vi "HandleObservationSync_002.vi"(8 "error in (no error)":errorcluster, 11 "S4GUI in":refnum<class "S4GUI.lvclass">) -> (0 "error out":errorcluster, 3 "S4GUI out":refnum<class "S4GUI.lvclass">)   [LabVIEW 2018, in "S4GUI.lvclass"] (continued)
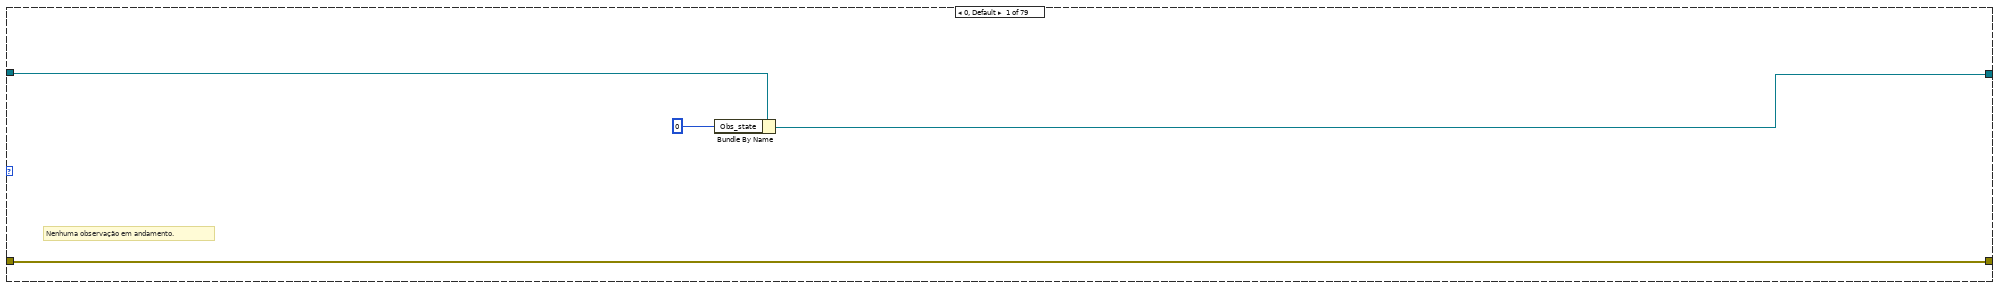
[diagram p2: hidden frame]
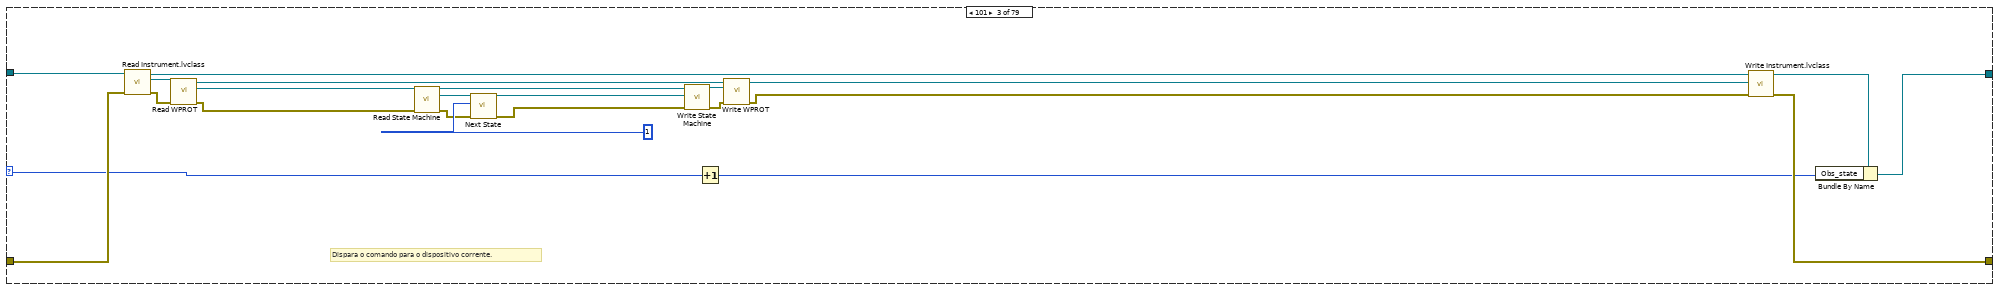
[diagram p4: hidden frame]
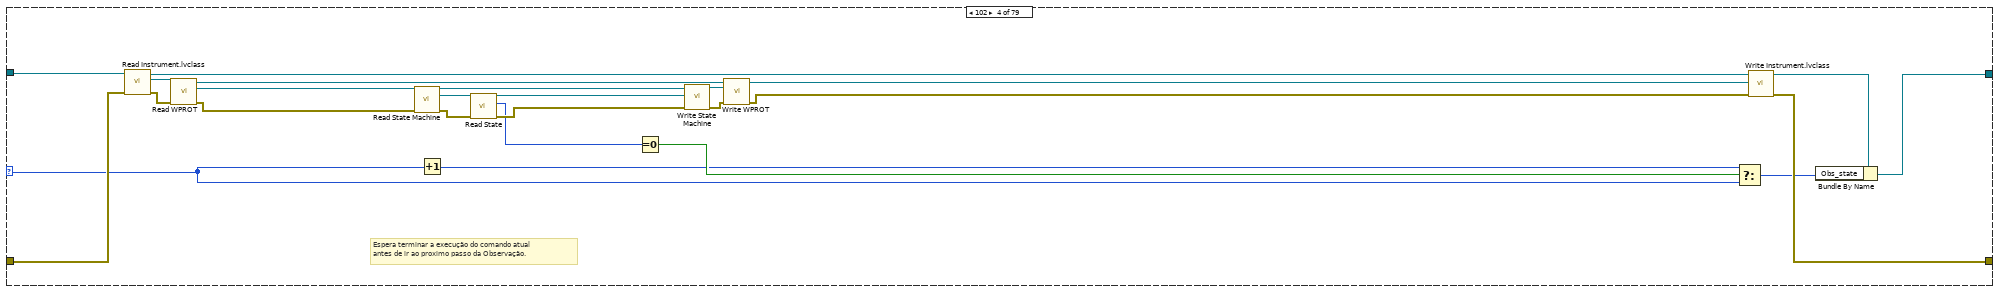
[diagram p5: hidden frame]
              n1811 = call-dynamic "Read Channel.vi"("error in (no error)"=w5159, "Acquisition in"=w5160) -> ("error out"=w5144:errorcluster, "Channel.lvclass"=w5146:refnum<class "Channel.lvclass">, "Acquisition out"=w5158:refnum<class "Acquisition.lvclass">)  [unwired: 7 in]
              n1812 = call-dynamic "Read wait_expose.vi"("error in (no error)"=w5144, "Channel in"=w5146) -> ("error out"=w5143:errorcluster, "wait_expose"=w5142:bool, "Channel out"=w5145:refnum<class "Channel.lvclass">)  [unwired: 7 in]
              n1813 = call-dynamic "Read State Machine.vi"("error in (no error)"=w5143, "Device in"=w5145) -> ("error out"=w5150:errorcluster, "State Machine.lvclass"=w5152:refnum<class "State Machine.lvclass">, "Device out"=w5154:refnum<class "Channel.lvclass">)  [unwired: 7 in]
              n1814 = call-dynamic "Read State.vi"("error in (no error)"=w5150, "State Machine in"=w5152) -> ("error out"=w5149:errorcluster, "State"=w5147:i32, "State Machine out"=w5151:refnum<class "State Machine.lvclass">)  [unwired: 7 in]
              n1815 = Equal To 0?(x=w5147) -> (x = 0?=w5148:bool)
              n1816 = call-dynamic "Write State Machine.vi"("error in (no error)"=w5149, "State Machine.lvclass"=w5151, "Device in"=w5154) -> ("error out"=w5153:errorcluster, "Device out"=w5155:refnum<class "Channel.lvclass">)  [unwired: 7 in]
              n1817 = call-dynamic "Write Channel.vi"("error in (no error)"=w5153, "Channel.lvclass"=w5155, "Acquisition in"=w5158) -> ("error out"=w5156:errorcluster, "Acquisition out"=w5157:refnum<class "Acquisition.lvclass">)  [unwired: 7 in]
            }
          }
          n1818 = call "Write AcquisitionB.vi"("error in (no error)"=w5080, "Acquisition.lvclass"=w5082, "S4ACS_GUI in"=w5081) -> ("error out"=w5076:errorcluster, "S4ACS_GUI out"=w5075:refnum<class "S4GUI.lvclass">)  [unwired: 7 in]
          n1819 = call-dynamic "Read AcquisitionC.vi"("error in (no error)"=w5076, "S4ACS_GUI in"=w5075) -> ("error out"=w5058:errorcluster, "Acquisition.lvclass"=w5060:refnum<class "Acquisition.lvclass">, "S4ACS_GUI out"=w5078:refnum<class "S4GUI.lvclass">)  [unwired: 7 in]
          n1820 = call-dynamic "Read enabled.vi"("error in (no error)"=w5058, "Server in"=w5060) -> ("error out"=w5057:errorcluster, "enabled"=w5056:bool, "Server out"=w5059:refnum<class "Acquisition.lvclass">)  [unwired: 7 in]
          n1821 = case shown="True" w5056 {
            tunnel: [w5117 w5132] -> w5079
            tunnel: [w5118 w5131] -> w5077
            tunnel: w5059 -> [w5118 w5127]
            tunnel: w5057 -> [w5117 w5126]
            tunnel: [TRUE w5124] -> w5045
            tunnel: [FALSE ("expose") w5119] -> w5041
            frame False {
            }
            frame True {
              n1822 = call-dynamic "Read Channel.vi"("error in (no error)"=w5126, "Acquisition in"=w5127) -> ("error out"=w5121:errorcluster, "Channel.lvclass"=w5123:refnum<class "Channel.lvclass">, "Acquisition out"=w5130:refnum<class "Acquisition.lvclass">)  [unwired: 7 in]
              n1823 = call-dynamic "Read wait_expose.vi"("error in (no error)"=w5121, "Channel in"=w5123) -> ("error out"=w5120:errorcluster, "wait_expose"=w5119:bool, "Channel out"=w5122:refnum<class "Channel.lvclass">)  [unwired: 7 in]
              n1824 = call-dynamic "Read State Machine.vi"("error in (no error)"=w5120, "Device in"=w5122) -> ("error out"=w5128:errorcluster, "State Machine.lvclass"=w5136:refnum<class "State Machine.lvclass">, "Device out"=w5134:refnum<class "Channel.lvclass">)  [unwired: 7 in]
              n1825 = call-dynamic "Read State.vi"("error in (no error)"=w5128, "State Machine in"=w5136) -> ("error out"=w5129:errorcluster, "State"=w5125:i32, "State Machine out"=w5137:refnum<class "State Machine.lvclass">)  [unwired: 7 in]
              n1826 = Equal To 0?(x=w5125) -> (x = 0?=w5124:bool)
              n1827 = call-dynamic "Write State Machine.vi"("error in (no error)"=w5129, "State Machine.lvclass"=w5137, "Device in"=w5134) -> ("error out"=w5135:errorcluster, "Device out"=w5133:refnum<class "Channel.lvclass">)  [unwired: 7 in]
              n1828 = call-dynamic "Write Channel.vi"("error in (no error)"=w5135, "Channel.lvclass"=w5133, "Acquisition in"=w5130) -> ("error out"=w5132:errorcluster, "Acquisition out"=w5131:refnum<class "Acquisition.lvclass">)  [unwired: 7 in]
            }
          }
          n1829 = call-dynamic "Write AcquisitionC.vi"("error in (no error)"=w5079, "Acquisition.lvclass"=w5077, "S4ACS_GUI in"=w5078) -> ("error out"=w5055:errorcluster, "S4ACS_GUI out"=w5071:refnum<class "S4GUI.lvclass">)  [unwired: 7 in]
          n1830 = call-dynamic "Read AcquisitionD.vi"("error in (no error)"=w5055, "S4ACS_GUI in"=w5071) -> ("error out"=w5051:errorcluster, "Acquisition.lvclass"=w5054:refnum<class "Acquisition.lvclass">, "S4ACS_GUI out"=w5073:refnum<class "S4GUI.lvclass">)  [unwired: 7 in]
          n1831 = call-dynamic "Read enabled.vi"("error in (no error)"=w5051, "Server in"=w5054) -> ("error out"=w5052:errorcluster, "enabled"=w5050:bool, "Server out"=w5053:refnum<class "Acquisition.lvclass">)  [unwired: 7 in]
          n1832 = case shown="True" w5050 {
            tunnel: [w5095 w5113] -> w5074
            tunnel: [w5094 w5112] -> w5072
            tunnel: [TRUE w5102] -> w5044
            tunnel: w5053 -> [w5095 w5104]
            tunnel: w5052 -> [w5094 w5103]
            tunnel: [FALSE ("expose") w5096] -> w5040
            frame False {
            }
            frame True {
              n1833 = call-dynamic "Read Channel.vi"("error in (no error)"=w5103, "Acquisition in"=w5104) -> ("error out"=w5098:errorcluster, "Channel.lvclass"=w5100:refnum<class "Channel.lvclass">, "Acquisition out"=w5114:refnum<class "Acquisition.lvclass">)  [unwired: 7 in]
              n1834 = call-dynamic "Read wait_expose.vi"("error in (no error)"=w5098, "Channel in"=w5100) -> ("error out"=w5097:errorcluster, "wait_expose"=w5096:bool, "Channel out"=w5099:refnum<class "Channel.lvclass">)  [unwired: 7 in]
              n1835 = call-dynamic "Read State Machine.vi"("error in (no error)"=w5097, "Device in"=w5099) -> ("error out"=w5106:errorcluster, "State Machine.lvclass"=w5108:refnum<class "State Machine.lvclass">, "Device out"=w5110:refnum<class "Channel.lvclass">)  [unwired: 7 in]
              n1836 = call-dynamic "Read State.vi"("error in (no error)"=w5106, "State Machine in"=w5108) -> ("error out"=w5105:errorcluster, "State"=w5101:i32, "State Machine out"=w5107:refnum<class "State Machine.lvclass">)  [unwired: 7 in]
              n1837 = Equal To 0?(x=w5101) -> (x = 0?=w5102:bool)
              n1838 = call-dynamic "Write State Machine.vi"("error in (no error)"=w5105, "State Machine.lvclass"=w5107, "Device in"=w5110) -> ("error out"=w5109:errorcluster, "Device out"=w5111:refnum<class "Channel.lvclass">)  [unwired: 7 in]
              n1839 = call-dynamic "Write Channel.vi"("error in (no error)"=w5109, "Channel.lvclass"=w5111, "Acquisition in"=w5114) -> ("error out"=w5112:errorcluster, "Acquisition out"=w5113:refnum<class "Acquisition.lvclass">)  [unwired: 7 in]
            }
          }
          n1840 = call-dynamic "Write AcquisitionD.vi"("error in (no error)"=w5072, "Acquisition.lvclass"=w5074, "S4ACS_GUI in"=w5073) -> ("error out"=w5038:errorcluster, "S4ACS_GUI out"=w5039:refnum<class "S4GUI.lvclass">)  [unwired: 7 in]
          n1841 = Compound Arithmetic op=OR(w5043, w5042, w5041, w5040) -> ()  [unwired: 1 out]
          n1842 = Compound Arithmetic op=AND(w5047, w5046, w5045, w5044) -> (w5048:bool)
          n1843 = Increment(x=w5049) -> (x+1=w5037:u32)
          n1844 = Select(t=w5037, s=w5048, f=w5049) -> (s? t:f=w5085:u32)
          n1845 = Bundle By Name(cluster=w5039, "Obs_state"=w5085) -> (w5086:refnum<class "S4GUI.lvclass">)
        }
        frame 364 {
          n1846 = flat-sequence {
            tunnel: [w5197] -> w5185
            tunnel: w5186 -> [w5197]
            tunnel: [w5193] -> w5184
            frame #0 {
              # "Espera 2s desde que enviou o comando\nWRITE_HEADER_DATA para os ACS"
              n1847 = local read "time9"() -> (w5192:u32)
              n1848 = Tick Count (ms)() -> (millisecond timer value=w5196:u32)
              "time 10" <- w5196
              n1849 = Subtract(x=w5196, y=w5192) -> (x-y=w5195:u32)
              "delay 89" <- w5195
              n1850 = Greater?(x=w5195, y=u32 2000) -> (0:w5193:bool)
            }
          }
          n1851 = Increment(x=w5189) -> (x+1=w5188:u32)
          n1852 = Select(t=w5188, s=w5184, f=w5189) -> (s? t:f=w5190:u32)
          n1853 = Bundle By Name(cluster=w5187, "Obs_state"=w5190) -> (w5191:refnum<class "S4GUI.lvclass">)
        }
        frame 365 {
          n1854 = call-dynamic "Read AcquisitionA.vi"("error in (no error)"=w5238, "S4ACS_GUI in"=w5239) -> ("error out"=w5214:errorcluster, "Acquisition.lvclass"=w5217:refnum<class "Acquisition.lvclass">, "S4ACS_GUI out"=w5241:refnum<class "S4GUI.lvclass">)  [unwired: 7 in]
          n1855 = call-dynamic "Read enabled.vi"("error in (no error)"=w5214, "Server in"=w5217) -> ("error out"=w5213:errorcluster, "enabled"=w5215:bool, "Server out"=w5216:refnum<class "Acquisition.lvclass">)  [unwired: 7 in]
          n1856 = case shown="True" w5215 {
            tunnel: w5216 -> [w5295 w5310]
            tunnel: w5213 -> [w5294 w5309]
            tunnel: [w5295 w5307] -> w5242
            tunnel: [w5294 w5306] -> w5240
            frame False {
            }
            frame True {
              n1857 = call-dynamic "Read Channel.vi"("error in (no error)"=w5309, "Acquisition in"=w5310) -> ("error out"=w5302:errorcluster, "Channel.lvclass"=w5301:refnum<class "Channel.lvclass">, "Acquisition out"=w5308:refnum<class "Acquisition.lvclass">)  [unwired: 7 in]
              n1858 = call-dynamic "Read State Machine.vi"("error in (no error)"=w5302, "Device in"=w5301) -> ("error out"=w5303:errorcluster, "State Machine.lvclass"=w5305:refnum<class "State Machine.lvclass">, "Device out"=w5299:refnum<class "Channel.lvclass">)  [unwired: 7 in]
              n1859 = call "Next State.vi"("error in (no error)"=w5303, "New_State"=50, "State Machine in"=w5305) -> ("error out"=w5296:errorcluster, "State Machine out"=w5297:refnum<class "State Machine.lvclass">)  [unwired: 7 in]
              n1860 = call-dynamic "Write State Machine.vi"("error in (no error)"=w5296, "State Machine.lvclass"=w5297, "Device in"=w5299) -> ("error out"=w5298:errorcluster, "Device out"=w5300:refnum<class "Channel.lvclass">)  [unwired: 7 in]
              n1861 = call-dynamic "Write Channel.vi"("error in (no error)"=w5298, "Channel.lvclass"=w5300, "Acquisition in"=w5308) -> ("error out"=w5306:errorcluster, "Acquisition out"=w5307:refnum<class "Acquisition.lvclass">)  [unwired: 7 in]
            }
          }
          n1862 = call-dynamic "Write AcquisitionA.vi"("error in (no error)"=w5240, "Acquisition.lvclass"=w5242, "S4ACS_GUI in"=w5241) -> ("error out"=w5233:errorcluster, "S4ACS_GUI out"=w5234:refnum<class "S4GUI.lvclass">)  [unwired: 7 in]
          n1863 = call "Read AcquisitionB.vi"("error in (no error)"=w5233, "S4ACS_GUI in"=w5234) -> ("error out"=w5210:errorcluster, "Acquisition.lvclass"=w5212:refnum<class "Acquisition.lvclass">, "S4ACS_GUI out"=w5231:refnum<class "S4GUI.lvclass">)  [unwired: 7 in]
          n1864 = call-dynamic "Read enabled.vi"("error in (no error)"=w5210, "Server in"=w5212) -> ("error out"=w5209:errorcluster, "enabled"=w5208:bool, "Server out"=w5211:refnum<class "Acquisition.lvclass">)  [unwired: 7 in]
          n1865 = case shown="True" w5208 {
            tunnel: w5211 -> [w5278 w5293]
            tunnel: w5209 -> [w5277 w5292]
            tunnel: [w5278 w5290] -> w5232
            tunnel: [w5277 w5289] -> w5230
            frame False {
            }
            frame True {
              n1866 = call-dynamic "Read Channel.vi"("error in (no error)"=w5292, "Acquisition in"=w5293) -> ("error out"=w5285:errorcluster, "Channel.lvclass"=w5284:refnum<class "Channel.lvclass">, "Acquisition out"=w5291:refnum<class "Acquisition.lvclass">)  [unwired: 7 in]
              n1867 = call-dynamic "Read State Machine.vi"("error in (no error)"=w5285, "Device in"=w5284) -> ("error out"=w5286:errorcluster, "State Machine.lvclass"=w5288:refnum<class "State Machine.lvclass">, "Device out"=w5282:refnum<class "Channel.lvclass">)  [unwired: 7 in]
              n1868 = call "Next State.vi"("error in (no error)"=w5286, "New_State"=50, "State Machine in"=w5288) -> ("error out"=w5279:errorcluster, "State Machine out"=w5280:refnum<class "State Machine.lvclass">)  [unwired: 7 in]
              n1869 = call-dynamic "Write State Machine.vi"("error in (no error)"=w5279, "State Machine.lvclass"=w5280, "Device in"=w5282) -> ("error out"=w5281:errorcluster, "Device out"=w5283:refnum<class "Channel.lvclass">)  [unwired: 7 in]
              n1870 = call-dynamic "Write Channel.vi"("error in (no error)"=w5281, "Channel.lvclass"=w5283, "Acquisition in"=w5291) -> ("error out"=w5289:errorcluster, "Acquisition out"=w5290:refnum<class "Acquisition.lvclass">)  [unwired: 7 in]
            }
          }
          n1871 = call "Write AcquisitionB.vi"("error in (no error)"=w5230, "Acquisition.lvclass"=w5232, "S4ACS_GUI in"=w5231) -> ("error out"=w5226:errorcluster, "S4ACS_GUI out"=w5225:refnum<class "S4GUI.lvclass">)  [unwired: 7 in]
          n1872 = call-dynamic "Read AcquisitionC.vi"("error in (no error)"=w5226, "S4ACS_GUI in"=w5225) -> ("error out"=w5205:errorcluster, "Acquisition.lvclass"=w5207:refnum<class "Acquisition.lvclass">, "S4ACS_GUI out"=w5228:refnum<class "S4GUI.lvclass">)  [unwired: 7 in]
          n1873 = call-dynamic "Read enabled.vi"("error in (no error)"=w5205, "Server in"=w5207) -> ("error out"=w5204:errorcluster, "enabled"=w5203:bool, "Server out"=w5206:refnum<class "Acquisition.lvclass">)  [unwired: 7 in]
          n1874 = case shown="True" w5203 {
            tunnel: [w5260 w5268] -> w5229
            tunnel: [w5261 w5267] -> w5227
            tunnel: w5206 -> [w5261 w5265]
            tunnel: w5204 -> [w5260 w5264]
            frame False {
            }
            frame True {
              n1875 = call-dynamic "Read Channel.vi"("error in (no error)"=w5264, "Acquisition in"=w5265) -> ("error out"=w5272:errorcluster, "Channel.lvclass"=w5273:refnum<class "Channel.lvclass">, "Acquisition out"=w5266:refnum<class "Acquisition.lvclass">)  [unwired: 7 in]
              n1876 = call-dynamic "Read State Machine.vi"("error in (no error)"=w5272, "Device in"=w5273) -> ("error out"=w5271:errorcluster, "State Machine.lvclass"=w5269:refnum<class "State Machine.lvclass">, "Device out"=w5275:refnum<class "Channel.lvclass">)  [unwired: 7 in]
              n1877 = call "Next State.vi"("error in (no error)"=w5271, "New_State"=50, "State Machine in"=w5269) -> ("error out"=w5263:errorcluster, "State Machine out"=w5262:refnum<class "State Machine.lvclass">)  [unwired: 7 in]
              n1878 = call-dynamic "Write State Machine.vi"("error in (no error)"=w5263, "State Machine.lvclass"=w5262, "Device in"=w5275) -> ("error out"=w5276:errorcluster, "Device out"=w5274:refnum<class "Channel.lvclass">)  [unwired: 7 in]
              n1879 = call-dynamic "Write Channel.vi"("error in (no error)"=w5276, "Channel.lvclass"=w5274, "Acquisition in"=w5266) -> ("error out"=w5268:errorcluster, "Acquisition out"=w5267:refnum<class "Acquisition.lvclass">)  [unwired: 7 in]
            }
          }
          n1880 = call-dynamic "Write AcquisitionC.vi"("error in (no error)"=w5229, "Acquisition.lvclass"=w5227, "S4ACS_GUI in"=w5228) -> ("error out"=w5223:errorcluster, "S4ACS_GUI out"=w5222:refnum<class "S4GUI.lvclass">)  [unwired: 7 in]
          n1881 = call-dynamic "Read AcquisitionD.vi"("error in (no error)"=w5223, "S4ACS_GUI in"=w5222) -> ("error out"=w5200:errorcluster, "Acquisition.lvclass"=w5202:refnum<class "Acquisition.lvclass">, "S4ACS_GUI out"=w5221:refnum<class "S4GUI.lvclass">)  [unwired: 7 in]
          n1882 = call-dynamic "Read enabled.vi"("error in (no error)"=w5200, "Server in"=w5202) -> ("error out"=w5199:errorcluster, "enabled"=w5198:bool, "Server out"=w5201:refnum<class "Acquisition.lvclass">)  [unwired: 7 in]
          n1883 = case shown="True" w5198 {
            tunnel: w5199 -> [w5243 w5259]
            tunnel: [w5243 w5258] -> w5224
            tunnel: w5201 -> [w5244 w5249]
            tunnel: [w5244 w5247] -> w5220
            frame False {
            }
            frame True {
              n1884 = call-dynamic "Read Channel.vi"("error in (no error)"=w5259, "Acquisition in"=w5249) -> ("error out"=w5254:errorcluster, "Channel.lvclass"=w5253:refnum<class "Channel.lvclass">, "Acquisition out"=w5248:refnum<class "Acquisition.lvclass">)  [unwired: 7 in]
              n1885 = call-dynamic "Read State Machine.vi"("error in (no error)"=w5254, "Device in"=w5253) -> ("error out"=w5255:errorcluster, "State Machine.lvclass"=w5257:refnum<class "State Machine.lvclass">, "Device out"=w5251:refnum<class "Channel.lvclass">)  [unwired: 7 in]
              n1886 = call "Next State.vi"("error in (no error)"=w5255, "New_State"=50, "State Machine in"=w5257) -> ("error out"=w5245:errorcluster, "State Machine out"=w5246:refnum<class "State Machine.lvclass">)  [unwired: 7 in]
              n1887 = call-dynamic "Write State Machine.vi"("error in (no error)"=w5245, "State Machine.lvclass"=w5246, "Device in"=w5251) -> ("error out"=w5250:errorcluster, "Device out"=w5252:refnum<class "Channel.lvclass">)  [unwired: 7 in]
              n1888 = call-dynamic "Write Channel.vi"("error in (no error)"=w5250, "Channel.lvclass"=w5252, "Acquisition in"=w5248) -> ("error out"=w5258:errorcluster, "Acquisition out"=w5247:refnum<class "Acquisition.lvclass">)  [unwired: 7 in]
            }
          }
          n1889 = call-dynamic "Write AcquisitionD.vi"("error in (no error)"=w5224, "Acquisition.lvclass"=w5220, "S4ACS_GUI in"=w5221) -> ("error out"=w5219:errorcluster, "S4ACS_GUI out"=w5218:refnum<class "S4GUI.lvclass">)  [unwired: 7 in]
          n1890 = Increment(x=w5237) -> (x+1=w5236:u32)
          n1891 = Bundle By Name(cluster=w5218, "Obs_state"=w5236) -> (w5235:refnum<class "S4GUI.lvclass">)
        }
        frame 366 {
          # "Espera todos os canais com CyclesDone=0"
          # "Espera todos os canais chegarem ao estado ACTIVE\n(estados 54 e 55 de Channel:Run.vi)."
          n1892 = call-dynamic "Read AcquisitionA.vi"("error in (no error)"=w5362, "S4ACS_GUI in"=w5363) -> ("error out"=w5341:errorcluster, "Acquisition.lvclass"=w5342:refnum<class "Acquisition.lvclass">, "S4ACS_GUI out"=w5365:refnum<class "S4GUI.lvclass">)  [unwired: 7 in]
          n1893 = call-dynamic "Read enabled.vi"("error in (no error)"=w5341, "Server in"=w5342) -> ("error out"=w5343:errorcluster, "enabled"=w5345:bool, "Server out"=w5344:refnum<class "Acquisition.lvclass">)  [unwired: 7 in]
          n1894 = case shown="True" w5345 {
            tunnel: [w5442 w5461] -> w5366
            tunnel: [w5441 w5460] -> w5364
            tunnel: w5344 -> [w5442 w5453]
            tunnel: w5343 -> [w5441 w5452]
            tunnel: [TRUE w5451] -> w5323
            tunnel: [u32 0 ("CyclesDone") w5443] -> w5315
            frame False {
            }
            frame True {
              n1895 = call-dynamic "Read Channel.vi"("error in (no error)"=w5452, "Acquisition in"=w5453) -> ("error out"=w5446:errorcluster, "Channel.lvclass"=w5447:refnum<class "Channel.lvclass">, "Acquisition out"=w5462:refnum<class "Acquisition.lvclass">)  [unwired: 7 in]
              n1896 = call-dynamic "Read CyclesDone.vi"("error in (no error)"=w5446, "Channel in"=w5447) -> ("error out"=w5444:errorcluster, "CyclesDone"=w5443:u32, "Channel out"=w5445:refnum<class "Channel.lvclass">)  [unwired: 7 in]
              n1897 = call-dynamic "Read State Machine.vi"("error in (no error)"=w5444, "Device in"=w5445) -> ("error out"=w5454:errorcluster, "State Machine.lvclass"=w5456:refnum<class "State Machine.lvclass">, "Device out"=w5458:refnum<class "Channel.lvclass">)  [unwired: 7 in]
              n1898 = call-dynamic "Read State.vi"("error in (no error)"=w5454, "State Machine in"=w5456) -> ("error out"=w5448:errorcluster, "State"=w5450:i32, "State Machine out"=w5455:refnum<class "State Machine.lvclass">)  [unwired: 7 in]
              n1899 = Greater?(x=w5450, y=53) -> (0:w5451:bool)
              n1900 = call-dynamic "Write State Machine.vi"("error in (no error)"=w5448, "State Machine.lvclass"=w5455, "Device in"=w5458) -> ("error out"=w5457:errorcluster, "Device out"=w5459:refnum<class "Channel.lvclass">)  [unwired: 7 in]
              n1901 = call-dynamic "Write Channel.vi"("error in (no error)"=w5457, "Channel.lvclass"=w5459, "Acquisition in"=w5462) -> ("error out"=w5460:errorcluster, "Acquisition out"=w5461:refnum<class "Acquisition.lvclass">)  [unwired: 7 in]
            }
          }
          n1902 = call-dynamic "Write AcquisitionA.vi"("error in (no error)"=w5364, "Acquisition.lvclass"=w5366, "S4ACS_GUI in"=w5365) -> ("error out"=w5358:errorcluster, "S4ACS_GUI out"=w5359:refnum<class "S4GUI.lvclass">)  [unwired: 7 in]
          n1903 = call "Read AcquisitionB.vi"("error in (no error)"=w5358, "S4ACS_GUI in"=w5359) -> ("error out"=w5338:errorcluster, "Acquisition.lvclass"=w5340:refnum<class "Acquisition.lvclass">, "S4ACS_GUI out"=w5356:refnum<class "S4GUI.lvclass">)  [unwired: 7 in]
          n1904 = call-dynamic "Read enabled.vi"("error in (no error)"=w5338, "Server in"=w5340) -> ("error out"=w5337:errorcluster, "enabled"=w5336:bool, "Server out"=w5339:refnum<class "Acquisition.lvclass">)  [unwired: 7 in]
          n1905 = case shown="True" w5336 {
            tunnel: w5339 -> [w5418 w5438]
            tunnel: w5337 -> [w5417 w5437]
            tunnel: [w5418 w5435] -> w5357
            tunnel: [w5417 w5434] -> w5355
            tunnel: [TRUE w5425] -> w5322
            tunnel: [u32 0 ("CyclesDone") w5419] -> w5316
            frame False {
            }
            frame True {
              n1906 = call-dynamic "Read Channel.vi"("error in (no error)"=w5437, "Acquisition in"=w5438) -> ("error out"=w5421:errorcluster, "Channel.lvclass"=w5423:refnum<class "Channel.lvclass">, "Acquisition out"=w5436:refnum<class "Acquisition.lvclass">)  [unwired: 7 in]
              n1907 = call-dynamic "Read CyclesDone.vi"("error in (no error)"=w5421, "Channel in"=w5423) -> ("error out"=w5420:errorcluster, "CyclesDone"=w5419:u32, "Channel out"=w5422:refnum<class "Channel.lvclass">)  [unwired: 7 in]
              n1908 = call-dynamic "Read State Machine.vi"("error in (no error)"=w5420, "Device in"=w5422) -> ("error out"=w5428:errorcluster, "State Machine.lvclass"=w5430:refnum<class "State Machine.lvclass">, "Device out"=w5432:refnum<class "Channel.lvclass">)  [unwired: 7 in]
              n1909 = call-dynamic "Read State.vi"("error in (no error)"=w5428, "State Machine in"=w5430) -> ("error out"=w5427:errorcluster, "State"=w5424:i32, "State Machine out"=w5429:refnum<class "State Machine.lvclass">)  [unwired: 7 in]
              n1910 = Greater?(x=w5424, y=53) -> (0:w5425:bool)
              n1911 = call-dynamic "Write State Machine.vi"("error in (no error)"=w5427, "State Machine.lvclass"=w5429, "Device in"=w5432) -> ("error out"=w5431:errorcluster, "Device out"=w5433:refnum<class "Channel.lvclass">)  [unwired: 7 in]
              n1912 = call-dynamic "Write Channel.vi"("error in (no error)"=w5431, "Channel.lvclass"=w5433, "Acquisition in"=w5436) -> ("error out"=w5434:errorcluster, "Acquisition out"=w5435:refnum<class "Acquisition.lvclass">)  [unwired: 7 in]
            }
          }
          n1913 = call "Write AcquisitionB.vi"("error in (no error)"=w5355, "Acquisition.lvclass"=w5357, "S4ACS_GUI in"=w5356) -> ("error out"=w5351:errorcluster, "S4ACS_GUI out"=w5350:refnum<class "S4GUI.lvclass">)  [unwired: 7 in]
          n1914 = call-dynamic "Read AcquisitionC.vi"("error in (no error)"=w5351, "S4ACS_GUI in"=w5350) -> ("error out"=w5333:errorcluster, "Acquisition.lvclass"=w5335:refnum<class "Acquisition.lvclass">, "S4ACS_GUI out"=w5353:refnum<class "S4GUI.lvclass">)  [unwired: 7 in]
          n1915 = call-dynamic "Read enabled.vi"("error in (no error)"=w5333, "Server in"=w5335) -> ("error out"=w5332:errorcluster, "enabled"=w5331:bool, "Server out"=w5334:refnum<class "Acquisition.lvclass">)  [unwired: 7 in]
          n1916 = case shown="True" w5331 {
            tunnel: [w5393 w5409] -> w5354
            tunnel: [w5394 w5408] -> w5352
            tunnel: w5334 -> [w5394 w5404]
            tunnel: w5332 -> [w5393 w5403]
            tunnel: [TRUE w5400] -> w5321
            tunnel: [u32 0 ("CyclesDone") w5395] -> w5314
            frame False {
            }
            frame True {
              n1917 = call-dynamic "Read Channel.vi"("error in (no error)"=w5403, "Acquisition in"=w5404) -> ("error out"=w5397:errorcluster, "Channel.lvclass"=w5399:refnum<class "Channel.lvclass">, "Acquisition out"=w5407:refnum<class "Acquisition.lvclass">)  [unwired: 7 in]
              n1918 = call-dynamic "Read CyclesDone.vi"("error in (no error)"=w5397, "Channel in"=w5399) -> ("error out"=w5396:errorcluster, "CyclesDone"=w5395:u32, "Channel out"=w5398:refnum<class "Channel.lvclass">)  [unwired: 7 in]
              n1919 = call-dynamic "Read State Machine.vi"("error in (no error)"=w5396, "Device in"=w5398) -> ("error out"=w5405:errorcluster, "State Machine.lvclass"=w5413:refnum<class "State Machine.lvclass">, "Device out"=w5411:refnum<class "Channel.lvclass">)  [unwired: 7 in]
              n1920 = call-dynamic "Read State.vi"("error in (no error)"=w5405, "State Machine in"=w5413) -> ("error out"=w5406:errorcluster, "State"=w5401:i32, "State Machine out"=w5414:refnum<class "State Machine.lvclass">)  [unwired: 7 in]
              n1921 = Greater?(x=w5401, y=53) -> (0:w5400:bool)
              n1922 = call-dynamic "Write State Machine.vi"("error in (no error)"=w5406, "State Machine.lvclass"=w5414, "Device in"=w5411) -> ("error out"=w5412:errorcluster, "Device out"=w5410:refnum<class "Channel.lvclass">)  [unwired: 7 in]
              n1923 = call-dynamic "Write Channel.vi"("error in (no error)"=w5412, "Channel.lvclass"=w5410, "Acquisition in"=w5407) -> ("error out"=w5409:errorcluster, "Acquisition out"=w5408:refnum<class "Acquisition.lvclass">)  [unwired: 7 in]
            }
          }
          n1924 = call-dynamic "Write AcquisitionC.vi"("error in (no error)"=w5354, "Acquisition.lvclass"=w5352, "S4ACS_GUI in"=w5353) -> ("error out"=w5330:errorcluster, "S4ACS_GUI out"=w5346:refnum<class "S4GUI.lvclass">)  [unwired: 7 in]
          n1925 = call-dynamic "Read AcquisitionD.vi"("error in (no error)"=w5330, "S4ACS_GUI in"=w5346) -> ("error out"=w5326:errorcluster, "Acquisition.lvclass"=w5329:refnum<class "Acquisition.lvclass">, "S4ACS_GUI out"=w5348:refnum<class "S4GUI.lvclass">)  [unwired: 7 in]
          n1926 = call-dynamic "Read enabled.vi"("error in (no error)"=w5326, "Server in"=w5329) -> ("error out"=w5327:errorcluster, "enabled"=w5325:bool, "Server out"=w5328:refnum<class "Acquisition.lvclass">)  [unwired: 7 in]
          n1927 = case shown="True" w5325 {
            tunnel: [w5370 w5389] -> w5349
            tunnel: [w5369 w5388] -> w5347
            tunnel: [TRUE w5377] -> w5320
            tunnel: w5328 -> [w5370 w5380]
            tunnel: w5327 -> [w5369 w5379]
            tunnel: [u32 0 ("CyclesDone") w5371] -> w5313
            frame False {
            }
            frame True {
              n1928 = call-dynamic "Read Channel.vi"("error in (no error)"=w5379, "Acquisition in"=w5380) -> ("error out"=w5373:errorcluster, "Channel.lvclass"=w5375:refnum<class "Channel.lvclass">, "Acquisition out"=w5390:refnum<class "Acquisition.lvclass">)  [unwired: 7 in]
              n1929 = call-dynamic "Read CyclesDone.vi"("error in (no error)"=w5373, "Channel in"=w5375) -> ("error out"=w5372:errorcluster, "CyclesDone"=w5371:u32, "Channel out"=w5374:refnum<class "Channel.lvclass">)  [unwired: 7 in]
              n1930 = call-dynamic "Read State Machine.vi"("error in (no error)"=w5372, "Device in"=w5374) -> ("error out"=w5382:errorcluster, "State Machine.lvclass"=w5384:refnum<class "State Machine.lvclass">, "Device out"=w5386:refnum<class "Channel.lvclass">)  [unwired: 7 in]
              n1931 = call-dynamic "Read State.vi"("error in (no error)"=w5382, "State Machine in"=w5384) -> ("error out"=w5381:errorcluster, "State"=w5376:i32, "State Machine out"=w5383:refnum<class "State Machine.lvclass">)  [unwired: 7 in]
              n1932 = Greater?(x=w5376, y=53) -> (0:w5377:bool)
              n1933 = call-dynamic "Write State Machine.vi"("error in (no error)"=w5381, "State Machine.lvclass"=w5383, "Device in"=w5386) -> ("error out"=w5385:errorcluster, "Device out"=w5387:refnum<class "Channel.lvclass">)  [unwired: 7 in]
              n1934 = call-dynamic "Write Channel.vi"("error in (no error)"=w5385, "Channel.lvclass"=w5387, "Acquisition in"=w5390) -> ("error out"=w5388:errorcluster, "Acquisition out"=w5389:refnum<class "Acquisition.lvclass">)  [unwired: 7 in]
            }
          }
          n1935 = call-dynamic "Write AcquisitionD.vi"("error in (no error)"=w5347, "Acquisition.lvclass"=w5349, "S4ACS_GUI in"=w5348) -> ("error out"=w5318:errorcluster, "S4ACS_GUI out"=w5319:refnum<class "S4GUI.lvclass">)  [unwired: 7 in]
          n1936 = Compound Arithmetic op=AND(w5323, w5322, w5321, w5320) -> ()  [unwired: 1 out]
          n1937 = Compound Arithmetic op=ADD(w5315, w5316, w5314, w5313) -> (w5312:u32)
          n1938 = Equal To 0?(x=w5312) -> (x = 0?=w5311:bool)
          n1939 = Increment(x=w5324) -> (x+1=w5317:u32)
          n1940 = Select(t=w5317, s=w5311, f=w5324) -> (s? t:f=w5360:u32)
          n1941 = Bundle By Name(cluster=w5319, "Obs_state"=w5360) -> (w5361:refnum<class "S4GUI.lvclass">)
        }
        frame 367 {
          # "T=canais receberam STOP"
          # "OV 2024.01.26 DEBUG - ignora os ciclos!!\nT= Todos os canais ativos no mesmo ciclo;\nF= Canais com ciclo diferente"
          # "T= Todos os canais ativos na mesma sequencia;\nF= Canais com sequencia diferente"
          # "Todos os CYCLES_DONE \nmudaram e são iguais?\nSe sim, avança a lâmina."
          n1942 = Unbundle By Name(w5498) -> ("cyclesDone"=w5492:u32)
          n1943 = call-dynamic "Read AcquisitionA.vi"("error in (no error)"=w5533, "S4ACS_GUI in"=w5498) -> ("error out"=w5513:errorcluster, "Acquisition.lvclass"=w5514:refnum<class "Acquisition.lvclass">, "S4ACS_GUI out"=w5535:refnum<class "S4GUI.lvclass">)  [unwired: 7 in]
          n1944 = call-dynamic "Read enabled.vi"("error in (no error)"=w5513, "Server in"=w5514) -> ("error out"=w5512:errorcluster, "enabled"=w5480:bool, "Server out"=w5511:refnum<class "Acquisition.lvclass">)  [unwired: 7 in]
          n1945 = case shown="True" w5480 {
            tunnel: w5512 -> [w5750 w5769]
            tunnel: [w5751 w5767] -> w5536
            tunnel: [w5750 w5766] -> w5534
            tunnel: [u32 0 ("SequesDone") w5765] -> w5486
            tunnel: w5511 -> [w5751 w5764]
            tunnel: w5492 -> [_ w5763]
            tunnel: [TRUE w5762] -> w5497
            tunnel: [u32 0 ("CubesDone") w5761] -> w5473
            tunnel: [FALSE ("stopping") w5752] -> w5469
            frame False {
            }
            frame True {
              # "CYCLES_DONE = 0->1"
              n1946 = call-dynamic "Read Channel.vi"("error in (no error)"=w5769, "Acquisition in"=w5764) -> ("error out"=w5758:errorcluster, "Channel.lvclass"=w5760:refnum<class "Channel.lvclass">, "Acquisition out"=w5768:refnum<class "Acquisition.lvclass">)  [unwired: 7 in]
              n1947 = call-dynamic "Read CyclesDone.vi"("error in (no error)"=w5758, "Channel in"=w5760) -> ("error out"=w5757:errorcluster, "CyclesDone"=w5761:u32, "Channel out"=w5759:refnum<class "Channel.lvclass">)  [unwired: 7 in]
              n1948 = call-dynamic "Read CyclesDone.vi"("error in (no error)"=w5757, "Channel in"=w5759) -> ("error out"=w5755:errorcluster, "CyclesDone"=w5765:u32, "Channel out"=w5756:refnum<class "Channel.lvclass">)  [unwired: 7 in]
              n1949 = Not Equal?(x=w5765, y=w5763) -> (x != y?=w5762:bool)
              n1950 = call-dynamic "Read stopping.vi"("error in (no error)"=w5755, "Channel in"=w5756) -> ("error out"=w5754:errorcluster, "stopping"=w5752:bool, "Channel out"=w5753:refnum<class "Channel.lvclass">)  [unwired: 7 in]
              n1951 = call-dynamic "Write Channel.vi"("error in (no error)"=w5754, "Channel.lvclass"=w5753, "Acquisition in"=w5768) -> ("error out"=w5766:errorcluster, "Acquisition out"=w5767:refnum<class "Acquisition.lvclass">)  [unwired: 7 in]
            }
          }
          n1952 = call-dynamic "Write AcquisitionA.vi"("error in (no error)"=w5534, "Acquisition.lvclass"=w5536, "S4ACS_GUI in"=w5535) -> ("error out"=w5530:errorcluster, "S4ACS_GUI out"=w5529:refnum<class "S4GUI.lvclass">)  [unwired: 7 in]
          n1953 = call "Read AcquisitionB.vi"("error in (no error)"=w5530, "S4ACS_GUI in"=w5529) -> ("error out"=w5507:errorcluster, "Acquisition.lvclass"=w5510:refnum<class "Acquisition.lvclass">, "S4ACS_GUI out"=w5531:refnum<class "S4GUI.lvclass">)  [unwired: 7 in]
          n1954 = call-dynamic "Read enabled.vi"("error in (no error)"=w5507, "Server in"=w5510) -> ("error out"=w5508:errorcluster, "enabled"=w5479:bool, "Server out"=w5509:refnum<class "Acquisition.lvclass">)  [unwired: 7 in]
          n1955 = case shown="True" w5479 {
            tunnel: w5508 -> [w5726 w5745]
            tunnel: w5509 -> [w5727 w5744]
            tunnel: [u32 0 ("SequesDone") w5739] -> w5483
            tunnel: [w5726 w5743] -> w5528
            tunnel: [w5727 w5742] -> w5527
            tunnel: w5492 -> [_ w5738]
            tunnel: [TRUE w5737] -> w5493
            tunnel: [u32 0 ("CubesDone") w5732] -> w5472
            tunnel: [FALSE ("stopping") w5728] -> w5468
            frame False {
            }
            frame True {
              n1956 = call-dynamic "Read Channel.vi"("error in (no error)"=w5745, "Acquisition in"=w5744) -> ("error out"=w5734:errorcluster, "Channel.lvclass"=w5736:refnum<class "Channel.lvclass">, "Acquisition out"=w5740:refnum<class "Acquisition.lvclass">)  [unwired: 7 in]
              n1957 = call-dynamic "Read CyclesDone.vi"("error in (no error)"=w5734, "Channel in"=w5736) -> ("error out"=w5733:errorcluster, "CyclesDone"=w5732:u32, "Channel out"=w5735:refnum<class "Channel.lvclass">)  [unwired: 7 in]
              n1958 = call-dynamic "Read CyclesDone.vi"("error in (no error)"=w5733, "Channel in"=w5735) -> ("error out"=w5730:errorcluster, "CyclesDone"=w5739:u32, "Channel out"=w5741:refnum<class "Channel.lvclass">)  [unwired: 7 in]
              n1959 = Not Equal?(x=w5739, y=w5738) -> (x != y?=w5737:bool)
              n1960 = call-dynamic "Read stopping.vi"("error in (no error)"=w5730, "Channel in"=w5741) -> ("error out"=w5729:errorcluster, "stopping"=w5728:bool, "Channel out"=w5731:refnum<class "Channel.lvclass">)  [unwired: 7 in]
              n1961 = call-dynamic "Write Channel.vi"("error in (no error)"=w5729, "Channel.lvclass"=w5731, "Acquisition in"=w5740) -> ("error out"=w5743:errorcluster, "Acquisition out"=w5742:refnum<class "Acquisition.lvclass">)  [unwired: 7 in]
            }
          }
          n1962 = Max & Min(x=w5473, y=w5472) -> (max(x,y)=w5489:u32)  [unwired: 1 out]
          n1963 = Max & Min(x=w5486, y=w5483) -> (max(x,y)=w5496:u32)  [unwired: 1 out]
          n1964 = call "Write AcquisitionB.vi"("error in (no error)"=w5528, "Acquisition.lvclass"=w5527, "S4ACS_GUI in"=w5531) -> ("error out"=w5520:errorcluster, "S4ACS_GUI out"=w5519:refnum<class "S4GUI.lvclass">)  [unwired: 7 in]
          n1965 = call-dynamic "Read AcquisitionC.vi"("error in (no error)"=w5520, "S4ACS_GUI in"=w5519) -> ("error out"=w5504:errorcluster, "Acquisition.lvclass"=w5506:refnum<class "Acquisition.lvclass">, "S4ACS_GUI out"=w5522:refnum<class "S4GUI.lvclass">)  [unwired: 7 in]
          n1966 = call-dynamic "Read enabled.vi"("error in (no error)"=w5504, "Server in"=w5506) -> ("error out"=w5503:errorcluster, "enabled"=w5478:bool, "Server out"=w5505:refnum<class "Acquisition.lvclass">)  [unwired: 7 in]
          n1967 = case shown="True" w5478 {
            tunnel: [w5702 w5721] -> w5523
            tunnel: [w5703 w5720] -> w5521
            tunnel: w5503 -> [w5702 w5717]
            tunnel: w5505 -> [w5703 w5718]
            tunnel: [u32 0 ("SequesDone") w5716] -> w5482
            tunnel: w5492 -> [_ w5715]
            tunnel: [TRUE w5714] -> w5491
            tunnel: [u32 0 ("CubesDone") w5708] -> w5471
            tunnel: [FALSE ("stopping") w5704] -> w5467
            frame False {
            }
            frame True {
              n1968 = call-dynamic "Read Channel.vi"("error in (no error)"=w5717, "Acquisition in"=w5718) -> ("error out"=w5710:errorcluster, "Channel.lvclass"=w5712:refnum<class "Channel.lvclass">, "Acquisition out"=w5719:refnum<class "Acquisition.lvclass">)  [unwired: 7 in]
              n1969 = call-dynamic "Read CyclesDone.vi"("error in (no error)"=w5710, "Channel in"=w5712) -> ("error out"=w5709:errorcluster, "CyclesDone"=w5708:u32, "Channel out"=w5711:refnum<class "Channel.lvclass">)  [unwired: 7 in]
              n1970 = call-dynamic "Read CyclesDone.vi"("error in (no error)"=w5709, "Channel in"=w5711) -> ("error out"=w5706:errorcluster, "CyclesDone"=w5716:u32, "Channel out"=w5713:refnum<class "Channel.lvclass">)  [unwired: 7 in]
              n1971 = Not Equal?(x=w5716, y=w5715) -> (x != y?=w5714:bool)
              n1972 = call-dynamic "Read stopping.vi"("error in (no error)"=w5706, "Channel in"=w5713) -> ("error out"=w5705:errorcluster, "stopping"=w5704:bool, "Channel out"=w5707:refnum<class "Channel.lvclass">)  [unwired: 7 in]
              n1973 = call-dynamic "Write Channel.vi"("error in (no error)"=w5705, "Channel.lvclass"=w5707, "Acquisition in"=w5719) -> ("error out"=w5721:errorcluster, "Acquisition out"=w5720:refnum<class "Acquisition.lvclass">)  [unwired: 7 in]
            }
          }
          n1974 = call-dynamic "Write AcquisitionC.vi"("error in (no error)"=w5523, "Acquisition.lvclass"=w5521, "S4ACS_GUI in"=w5522) -> ("error out"=w5517:errorcluster, "S4ACS_GUI out"=w5518:refnum<class "S4GUI.lvclass">)  [unwired: 7 in]
          n1975 = call-dynamic "Read AcquisitionD.vi"("error in (no error)"=w5517, "S4ACS_GUI in"=w5518) -> ("error out"=w5500:errorcluster, "Acquisition.lvclass"=w5502:refnum<class "Acquisition.lvclass">, "S4ACS_GUI out"=w5524:refnum<class "S4GUI.lvclass">)  [unwired: 7 in]
          n1976 = call-dynamic "Read enabled.vi"("error in (no error)"=w5500, "Server in"=w5502) -> ("error out"=w5499:errorcluster, "enabled"=w5477:bool, "Server out"=w5501:refnum<class "Acquisition.lvclass">)  [unwired: 7 in]
          n1977 = Build Array(w5480, w5479, w5478, w5477) -> (w5476:bool[])
          n1978 = case shown="True" w5477 {
            tunnel: [w5679 w5697] -> w5526
            tunnel: [w5678 w5696] -> w5525
            tunnel: w5501 -> [w5679 w5695]
            tunnel: w5499 -> [w5678 w5694]
            tunnel: [u32 0 ("SequesDone") w5692] -> w5485
            tunnel: w5492 -> [_ w5691]
            tunnel: [TRUE w5690] -> w5490
            tunnel: [u32 0 ("CubesDone") w5684] -> w5470
            tunnel: [FALSE ("stopping") w5680] -> w5466
            frame False {
            }
            frame True {
              n1979 = call-dynamic "Read Channel.vi"("error in (no error)"=w5694, "Acquisition in"=w5695) -> ("error out"=w5686:errorcluster, "Channel.lvclass"=w5688:refnum<class "Channel.lvclass">, "Acquisition out"=w5693:refnum<class "Acquisition.lvclass">)  [unwired: 7 in]
              n1980 = call-dynamic "Read CyclesDone.vi"("error in (no error)"=w5686, "Channel in"=w5688) -> ("error out"=w5685:errorcluster, "CyclesDone"=w5684:u32, "Channel out"=w5687:refnum<class "Channel.lvclass">)  [unwired: 7 in]
              n1981 = call-dynamic "Read CyclesDone.vi"("error in (no error)"=w5685, "Channel in"=w5687) -> ("error out"=w5682:errorcluster, "CyclesDone"=w5692:u32, "Channel out"=w5689:refnum<class "Channel.lvclass">)  [unwired: 7 in]
              n1982 = Not Equal?(x=w5692, y=w5691) -> (x != y?=w5690:bool)
              n1983 = call-dynamic "Read stopping.vi"("error in (no error)"=w5682, "Channel in"=w5689) -> ("error out"=w5681:errorcluster, "stopping"=w5680:bool, "Channel out"=w5683:refnum<class "Channel.lvclass">)  [unwired: 7 in]
              n1984 = call-dynamic "Write Channel.vi"("error in (no error)"=w5681, "Channel.lvclass"=w5683, "Acquisition in"=w5693) -> ("error out"=w5696:errorcluster, "Acquisition out"=w5697:refnum<class "Acquisition.lvclass">)  [unwired: 7 in]
            }
          }
          n1985 = Boolean Array To Number(Boolean array=w5476) -> (number=w5474:u32)
          n1986 = Max & Min(x=w5471, y=w5470) -> (max(x,y)=w5488:u32)  [unwired: 1 out]
          n1987 = Max & Min(x=w5482, y=w5485) -> (max(x,y)=w5495:u32)  [unwired: 1 out]
          n1988 = Compound Arithmetic op=AND(w5497, w5493, w5491, w5490) -> (w5475:bool)
          n1989 = Max & Min(x=w5496, y=w5495) -> (max(x,y)=w5494:u32)  [unwired: 1 out]
          n1990 = Max & Min(x=w5489, y=w5488) -> (max(x,y)=w5487:u32)  [unwired: 1 out]
          n1991 = case shown="12" w5474 {
            tunnel: w5473 -> [w5544 _ w5556 _ w5565 _ w5571 w5577 _ w5583 w5586 _]
            tunnel: w5470 -> [w5543 w5547 w5552 w5559 w5560 w5568 w5570 _ _ _ _ _]
            tunnel: w5472 -> [w5542 w5545 _ _ w5564 w5566 _ w5576 w5580 _ w5585 _]
            tunnel: w5471 -> [w5541 w5546 w5551 w5557 _ _ _ w5575 w5579 w5582 _ _]
            tunnel: [w5537 w5548 w5553 w5558 w5561 w5567 w5569 w5572 w5578 w5581 w5584 TRUE] -> _
            frame 15 {
              # "A,B,C,D ativos"
              n1992 = Equal?(x=w5544, y=w5542) -> (x = y?=w5540:bool)
              n1993 = Equal?(x=w5541, y=w5543) -> (x = y?=w5538:bool)
              n1994 = Equal?(x=w5542, y=w5541) -> (x = y?=w5539:bool)
              n1995 = Compound Arithmetic op=AND(w5540, w5539, w5538) -> (w5537:bool)
            }
            frame 14 {
              # "B,C e,D ativos"
              n1996 = Equal?(x=w5545, y=w5546) -> (x = y?=w5550:bool)
              n1997 = Equal?(x=w5546, y=w5547) -> (x = y?=w5549:bool)
              n1998 = Compound Arithmetic op=AND(w5550, w5549) -> (w5548:bool)
            }
            frame 13 {
              # "A,C e,D ativos"
              n1999 = Equal?(x=w5556, y=w5551) -> (x = y?=w5555:bool)
              n2000 = Equal?(x=w5551, y=w5552) -> (x = y?=w5554:bool)
              n2001 = Compound Arithmetic op=AND(w5555, w5554) -> (w5553:bool)
            }
            frame 12 {
              # "Só C e D ativos"
              n2002 = Equal?(x=w5557, y=w5559) -> (x = y?=w5558:bool)
            }
            frame 11 {
              # "A,B e,D ativos"
              n2003 = Equal?(x=w5565, y=w5564) -> (x = y?=w5563:bool)
              n2004 = Equal?(x=w5564, y=w5560) -> (x = y?=w5562:bool)
              n2005 = Compound Arithmetic op=AND(w5563, w5562) -> (w5561:bool)
            }
            frame 10 {
              # "Só B e D ativos"
              n2006 = Equal?(x=w5566, y=w5568) -> (x = y?=w5567:bool)
            }
            frame 9 {
              # "Só A e D ativos"
              n2007 = Equal?(x=w5571, y=w5570) -> (x = y?=w5569:bool)
            }
            frame 7 {
              # "A,B,C ativos"
              n2008 = Equal?(x=w5577, y=w5576) -> (x = y?=w5574:bool)
              n2009 = Equal?(x=w5576, y=w5575) -> (x = y?=w5573:bool)
              n2010 = Compound Arithmetic op=AND(w5574, w5573) -> (w5572:bool)
            }
            frame 6 {
              # "Só B e C ativos"
              n2011 = Equal?(x=w5580, y=w5579) -> (x = y?=w5578:bool)
            }
            frame 5 {
              # "Só A e C ativos"
              n2012 = Equal?(x=w5583, y=w5582) -> (x = y?=w5581:bool)
            }
            frame 3 {
              # "só A e B ativos"
              n2013 = Equal?(x=w5586, y=w5585) -> (x = y?=w5584:bool)
            }
            frame 0..2, 4, 8, Default {
              # "nenhum ou só 1  \ncanal ativo."
            }
          }
          n2014 = Compound Arithmetic op=OR(w5469, w5468, w5467, w5466) -> (w5465:bool)
          n2015 = case shown="0..2, 4, 8, Default" w5474 {
            tunnel: w5486 -> [w5595 _ w5607 _ w5616 _ w5622 w5628 _ w5634 w5637 _]
            tunnel: w5485 -> [w5594 w5598 w5603 w5610 w5611 w5619 w5621 _ _ _ _ _]
            tunnel: w5483 -> [w5593 w5596 _ _ w5615 w5617 _ w5627 w5631 _ w5636 _]
            tunnel: w5482 -> [w5592 w5597 w5602 w5608 _ _ _ w5626 w5630 w5633 _ _]
            tunnel: [w5588 w5599 w5604 w5609 w5612 w5618 w5620 w5623 w5629 w5632 w5635 TRUE] -> w5481
            frame 15 {
              # "A,B,C,D ativos"
              n2016 = Equal?(x=w5595, y=w5593) -> (x = y?=w5591:bool)
              n2017 = Equal?(x=w5592, y=w5594) -> (x = y?=w5589:bool)
              n2018 = Equal?(x=w5593, y=w5592) -> (x = y?=w5590:bool)
              n2019 = Compound Arithmetic op=AND(w5591, w5590, w5589) -> (w5588:bool)
            }
            frame 14 {
              # "B,C e,D ativos"
              n2020 = Equal?(x=w5596, y=w5597) -> (x = y?=w5601:bool)
              n2021 = Equal?(x=w5597, y=w5598) -> (x = y?=w5600:bool)
              n2022 = Compound Arithmetic op=AND(w5601, w5600) -> (w5599:bool)
            }
            frame 13 {
              # "A,C e,D ativos"
              n2023 = Equal?(x=w5607, y=w5602) -> (x = y?=w5606:bool)
              n2024 = Equal?(x=w5602, y=w5603) -> (x = y?=w5605:bool)
              n2025 = Compound Arithmetic op=AND(w5606, w5605) -> (w5604:bool)
            }
            frame 12 {
              # "Só C e D ativos"
              n2026 = Equal?(x=w5608, y=w5610) -> (x = y?=w5609:bool)
            }
            frame 11 {
              # "A,B e,D ativos"
              n2027 = Equal?(x=w5616, y=w5615) -> (x = y?=w5614:bool)
              n2028 = Equal?(x=w5615, y=w5611) -> (x = y?=w5613:bool)
              n2029 = Compound Arithmetic op=AND(w5614, w5613) -> (w5612:bool)
            }
            frame 10 {
              # "Só B e D ativos"
              n2030 = Equal?(x=w5617, y=w5619) -> (x = y?=w5618:bool)
            }
            frame 9 {
              # "Só A e D ativos"
              n2031 = Equal?(x=w5622, y=w5621) -> (x = y?=w5620:bool)
            }
            frame 7 {
              # "A,B,C ativos"
              n2032 = Equal?(x=w5628, y=w5627) -> (x = y?=w5625:bool)
              n2033 = Equal?(x=w5627, y=w5626) -> (x = y?=w5624:bool)
              n2034 = Compound Arithmetic op=AND(w5625, w5624) -> (w5623:bool)
            }
            frame 6 {
              # "Só B e C ativos"
              n2035 = Equal?(x=w5631, y=w5630) -> (x = y?=w5629:bool)
            }
            frame 5 {
              # "Só A e C ativos"
              n2036 = Equal?(x=w5634, y=w5633) -> (x = y?=w5632:bool)
            }
            frame 3 {
              # "só A e B ativos"
              n2037 = Equal?(x=w5637, y=w5636) -> (x = y?=w5635:bool)
            }
            frame 0..2, 4, 8, Default {
              # "nenhum ou só 1  \ncanal ativo."
            }
          }
          n2038 = call-dynamic "Write AcquisitionD.vi"("error in (no error)"=w5525, "Acquisition.lvclass"=w5526, "S4ACS_GUI in"=w5524) -> ("error out"=w5515:errorcluster, "S4ACS_GUI out"=w5516:refnum<class "S4GUI.lvclass">)  [unwired: 7 in]
          n2039 = And(x=w5475, y=w5481) -> (x .and. y?=w5484:bool)
          n2040 = case shown="True" w5484 {
            tunnel: w5516 -> [w5640 w5652]
            tunnel: [w5639 w5651] -> w5532
            tunnel: w5494 -> [_ w5650]
            tunnel: w5487 -> [_ _]
            tunnel: w5475 -> [w5641 _]
            tunnel: TRUE -> [_ w5649]
            tunnel: w5465 -> [_ w5648]
            tunnel: w5463 -> [_ w5647]
            frame False {
              n2041 = case shown="True" w5641 {
                tunnel: w5640 -> [w5642 w5646]
                tunnel: [w5642 w5645] -> w5639
                frame False {
                }
                frame True {
                  n2042 = Bundle By Name(cluster=w5646, "Obs_state"=u32 1, "Error Msg"="ERROR: Sequence_done not equal in all active channels.") -> (w5645:refnum<class "S4GUI.lvclass">)
                }
              }
            }
            frame True {
              n2043 = case shown="True" w5649 {
                tunnel: w5652 -> [w5654 w5664]
                tunnel: [w5653 w5663] -> w5651
                tunnel: w5650 -> [_ w5662]
                tunnel: w5648 -> [_ w5658]
                tunnel: w5647 -> [_ w5657]
                frame False {
                  n2044 = Bundle By Name(cluster=w5654, "Obs_state"=u32 1, "Error Msg"="ERROR: Cycles_done not equal in all active channels.") -> (w5653:refnum<class "S4GUI.lvclass">)
                }
                frame True {
                  # "STOP?"
                  n2045 = local read "time308"() -> (w5660:u32)
                  n2046 = Tick Count (ms)() -> (millisecond timer value=w5661:u32)
                  n2047 = Subtract(x=w5661, y=w5660) -> (x-y=→"delay Acq 2":u32)
                  n2048 = case shown="False" w5658 {
                    tunnel: w5664 -> [w5668 w5673]
                    tunnel: [w5667 w5672] -> w5663
                    tunnel: w5662 -> [w5665 w5669]
                    tunnel: w5657 -> [_ w5671]
                    frame True {
                      n2049 = Bundle By Name(cluster=w5668, "Obs_state"=u32 0, "sequesDone"=w5665, "cyclesDone"=w5665) -> (w5667:refnum<class "S4GUI.lvclass">)
                    }
                    frame False {
                      n2050 = Increment(x=w5671) -> (x+1=w5670:u32)
                      n2051 = Bundle By Name(cluster=w5673, "Obs_state"=w5670, "sequesDone"=w5669, "cyclesDone"=w5669) -> (w5672:refnum<class "S4GUI.lvclass">)
                    }
                  }
                }
              }
            }
          }
        }
        frame 368 {
          n2052 = Unbundle By Name(w5775) -> ("TelFocus.lvclass"=w5774:refnum<class "TelFocus.lvclass">)
          n2053 = call-dynamic "VerifSteps.vi"("error in (no error)"=w5771, "TelFocus in"=w5774) -> ("error out"=w5770:errorcluster, "continua?"=w5776:bool, "TelFocus out"=w5773:refnum<class "TelFocus.lvclass">)  [unwired: 7 in]
          n2054 = Bundle By Name(cluster=w5775, "TelFocus.lvclass"=w5773) -> (w5772:refnum<class "S4GUI.lvclass">)
          n2055 = Select(t=u32 360, s=w5776, f=u32 0) -> (s? t:f=w5779:u32)
          n2056 = Bundle By Name(cluster=w5772, "Obs_state"=w5779) -> (w5780:refnum<class "S4GUI.lvclass">)
        }
        frame 400 {
          # "Estado de \"Pause\": fica parado aqui até o botão START seja pressionado."
        }
        frame 500 {
          # "Espera terminar o envio de RESUME para todos os ACS."
          # "Estado de \"Pause\": fica parado aqui até o botão START seja pressionado."
          n2057 = call-dynamic "VerifyAcqIdle.vi"("error in (no error)"=w5785, "S4GUI in"=w5789) -> ("error out"=w5784:errorcluster, "idle"=w5788:bool, "S4GUI out"=w5787:refnum<class "S4GUI.lvclass">)  [unwired: 7 in]
          n2058 = case shown="True" w5788 {
            tunnel: w5787 -> [w5791 w5801]
            tunnel: [w5791 w5793] -> w5786
            tunnel: w5784 -> [w5790 w5800]
            tunnel: [w5790 w5794] -> w5783
            frame False {
            }
            frame True {
              n2059 = call-dynamic "LoadPrevAcqRunState.vi"("error in (no error)"=w5800, "S4GUI in"=w5801) -> ("error out"=w5795:errorcluster, "S4GUI out"=w5796:refnum<class "S4GUI.lvclass">)  [unwired: 8 in]
              n2060 = Tick Count (ms)() -> (millisecond timer value=w5792:u32)
              n2061 = call-dynamic "Read Obs_prevstate.vi"("error in (no error)"=w5795, "S4ACS_GUI in"=w5796) -> ("error out"=w5799:errorcluster, "Obs_prevstate"=w5797:u32, "S4ACS_GUI out"=w5798:refnum<class "S4GUI.lvclass">)  [unwired: 7 in]
              n2062 = local write "time307"(w5792) -> ()
              n2063 = local write "time1"(w5792) -> ()
              n2064 = call-dynamic "Write Obs_state.vi"("error in (no error)"=w5799, "Obs_state"=w5797, "S4ACS_GUI in"=w5798) -> ("error out"=w5794:errorcluster, "S4ACS_GUI out"=w5793:refnum<class "S4GUI.lvclass">)  [unwired: 7 in]
            }
          }
        }
      }
    }
    frame Error {
    }
  }
  "error out" <- w3
  "S4GUI out" <- w2
